vi "Detect Header.vi"(0 "read bit status":T1, 5 "header size":u8) -> (4 "header valid":bool)   [LabVIEW 2013, in "DIO SPI User Library.lvlib"]
doc: "This VI simply detects when all header bits have been read by the SPI slave. This detection allows data to be returned by the user logic registers in the case of a SPI read transaction."
uses:
  DIO SPI User Library.lvlib
  Perforce/MI/Apps/IP/SPI/trunk/1.1/source/LV/user.lib/._NI SPI IP/FPGA/Controllers/Public/Read Bit Status.ctl
panel:
  # "This VI simply detects when all header bits have been read by the SPI slave. This detection allows data to be returned by the user logic registers in the case of a SPI read transaction."
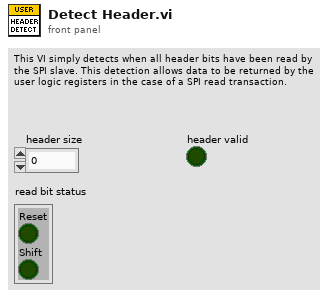
[diagram p1: front panel]
types:
  T1 = typedef "DIO SPI FPGA.lvlib/Read Bit Status.ctl" = cluster{"Reset":bool, "Shift":bool}
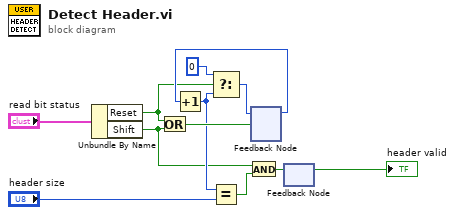
[diagram p0: block diagram]
diagram:
  n1 = Unbundle By Name("read bit status") -> ("Reset"=w5:bool, "Shift"=w1:bool)
  n2 = Or(x=w5, y=w1) -> (x .or. y?=w10:bool)
  n3 = feedback #1() -> (w9:u8)  [unwired: 1 in]
  n4 = Increment(x=w9) -> (x+1=w3:u8)
  n5 = Select(t=u8 0, s=w5, f=w3) -> (s? t:f=w11:u8)
  n6 = Equal?(x=w3, y="header size") -> (x = y?=w2:bool)
  n7 = And(x=w1, y=w2) -> (x .and. y?=w8:bool)
  n8 = feedback-in #1(w11, w10) -> ()
  n9 = feedback #2() -> (→"header valid":bool)  [unwired: 1 in]
  n10 = feedback-in #2(w8) -> ()
